vi "Import Bitfile Scalars.vi"   [LabVIEW 2018, in "Scripting API.lvlib"]
uses:
  Scripting API.lvlib
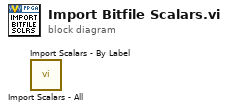
[diagram p0: block diagram]
diagram:
  n1 = call "Import Scalars - All.vi"() -> ()  [unwired: 9 in, 3 out]
  n2 = call "Import Scalars - By Label.vi"() -> ()  [unwired: 9 in, 3 out]
